vi "Render.vi"(8 "error in (no error)":errorcluster, 10 "String in":string, 11 "Paragraph in":refnum<class "Paragraph.lvclass">) -> (0 "error out":errorcluster, 2 "String out":string, 3 "Paragraph out":refnum<class "Paragraph.lvclass">)   [LabVIEW 2021, in "LvMarkdown.lvlib" / "Paragraph.lvclass"]
uses:
  Paragraph.lvclass
  C:/GitHub/LvMarkdown/src/LvMarkdown/Markdown.lvclass
  Paragraph.lvclass/Paragraph.ctl
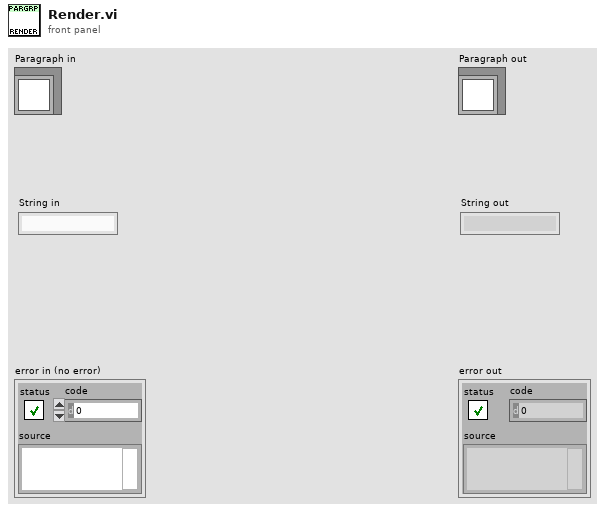
[diagram p1: front panel]
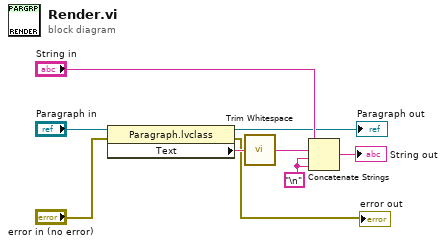
[diagram p0: block diagram]
diagram:
  w3 = "\n"
  n1 = property class="Paragraph.lvclass"(reference="Paragraph in", error in="error in (no error)") -> (reference out=→"Paragraph out":refnum<class "Paragraph.lvclass">, error out=→"error out":errorcluster, "Text"=w9:string)
  n2 = call <vilib>:"Trim Whitespace.vi"("string"=w9) -> ("trimmed string"=w8:string)  [unwired: 1 in]
  n3 = Concatenate Strings("String in", w8, w3, w3) -> (→"String out":string)
